vi "Test gRPC cRIO Read Raw Frame.vi"(11 "Test Case In":refnum<class "Test NI9862.lvclass">) -> (0 "error out":errorcluster, 3 "Test Case Out":refnum<class "Test NI9862.lvclass">)   [LabVIEW 2024, in "Test NI9862.lvclass"]
uses:
  Test NI9862.lvclass
  Source/Interfaces/IMessage/IMessage.lvclass
  Source/Configure Strategies/gRPC XNET Read Raw CAN Frame Strategy/gRPC XNET Read Raw CAN Frame Strategy.lvclass
  Source/Config from JSON/Config from JSON.lvclass
  Source/NI9862/NI9862.lvclass
  Test NI9862.lvclass/Test NI9862.ctl
  <vilib>/Astemes/LUnit/Test Case.lvclass
panel:
  out "Error Out":errorcluster
  out "Messages":refnum<class "IMessage.lvclass">[](array[class])
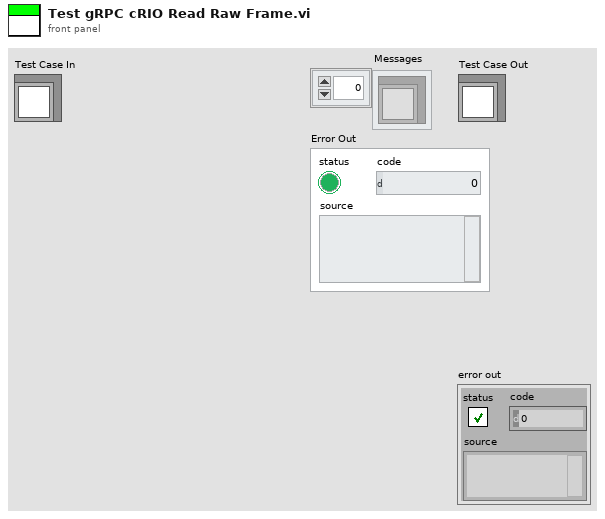
[diagram p1: front panel]
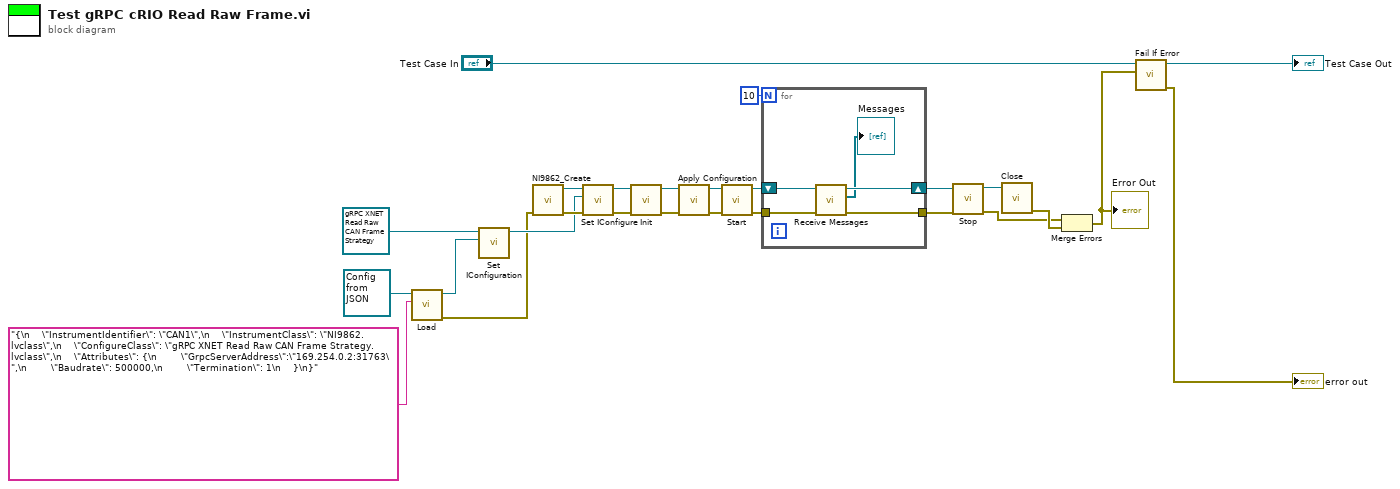
[diagram p0: block diagram]
diagram:
  n1 = call-dynamic "Load.vi"("Source"="{\n    \"InstrumentIdentifier\": \"CAN1\",\n    \"InstrumentClass\": \"NI9862.lvclass\",\n    \"ConfigureClass\": \"gRPC XNET Read Raw CAN Frame Strategy.lvclass\",\n    \"Attributes\": {\n        \"GrpcServerAddress\":\"169.254.0.2:31763\",\n        \"Baudrate\": 500000,\n        \"Termination\": 1\n    }\n}", "Config From JSON in"=refnum<class "Config from JSON.lvclass"> refnum ("Config from JSON.lvclass")) -> ("error out"=w4:errorcluster, "Config From JSON out"=w18:refnum<class "Config from JSON.lvclass">)  [unwired: 8 in]
  n2 = call-dynamic "Set IConfiguration.vi"("IConfiguration"=w18, "gRPC XNET Read Raw CAN Frame Strategy in"=refnum<class "gRPC XNET Read Raw CAN Frame Strategy.lvclass"> refnum ("IConfigure")) -> ("gRPC XNET Read Raw CAN Frame Strategy out"=w22:refnum<class "gRPC XNET Read Raw CAN Frame Strategy.lvclass">)  [unwired: 9 in]
  n3 = call "NI9862_Create.vi"("Error In"=w4) -> ("Error Out"=w23:errorcluster, "NI9862 out"=w9:refnum<class "NI9862.lvclass">)  [unwired: 9 in]
  n4 = call-dynamic "Set IConfigure.vi"("Error In"=w23, "IConfigure"=w22, "reference in"=w9) -> ("Error Out"=w17:errorcluster, "reference out"=w16:refnum<class "NI9862.lvclass">)  [unwired: 7 in]
  n5 = call-dynamic "Init.vi"("Error In"=w17, "reference in"=w16) -> ("Error Out"=w15:errorcluster, "reference out"=w14:refnum<class "NI9862.lvclass">)  [unwired: 8 in]
  n6 = call-dynamic "Apply Configuration.vi"("Error In"=w15, "reference in"=w14) -> ("Error Out"=w5:errorcluster, "reference out"=w6:refnum<class "NI9862.lvclass">)  [unwired: 8 in]
  n7 = call-dynamic "Start.vi"("Error In"=w5, "reference in"=w6) -> ("Error Out"=w11:errorcluster, "reference out"=w12:refnum<class "NI9862.lvclass">)  [unwired: 8 in]
  n8 = for {
    N: 10 -> [_]
    tunnel: w11 -> [w30]
    shift-right: [w29] -> w10
    shift-left: w12 -> [w31]
    tunnel: [w28] -> w8
    n9 = call-dynamic "Receive Messages.vi"("Error In"=w30, "reference in"=w31) -> ("Error Out"=w28:errorcluster, "Messages"=→"Messages":refnum<class "IMessage.lvclass">[], "reference out"=w29:refnum<class "NI9862.lvclass">)  [unwired: 7 in]
  }
  n10 = call-dynamic "Stop.vi"("Error In"=w8, "reference in"=w10) -> ("Error Out"=w1:errorcluster, "reference out"=w7:refnum<class "NI9862.lvclass">)  [unwired: 8 in]
  n11 = call-dynamic "Close.vi"("reference in"=w7) -> ("Error Out"=w3:errorcluster)  [unwired: 9 in, 1 out]
  n12 = Merge Errors(w1, w3) -> (w2:errorcluster)
  "Error Out" <- w2
  n13 = call <vilib>:"Fail If Error.vi"("Assert error"=w2, "LUnit Test Case In"="Test Case In") -> ("error out"=→"error out":errorcluster, "LUnit Test Case Out"=→"Test Case Out":refnum<class "Test NI9862.lvclass">)  [unwired: 8 in]
